vi "TreeEditor.vi"() -> ()   [LabVIEW 2016]
uses:
  ClassDataTree/ClassDataTree.lvclass
panel:
  in  "CreateChild":bool
  in  "LoadToFile":bool
  in  "SaveToFile":bool
  in  "Delete":bool
  in  "Update":bool
  in  "CreateTag":bool
  out "ClassDataTree":refnum<class "ClassDataTree.lvclass">
  in  "ExitApplocation":bool
  out "error out":errorcluster
  in  "CreateNameTag":string
  in  "Tree":string[](tree)
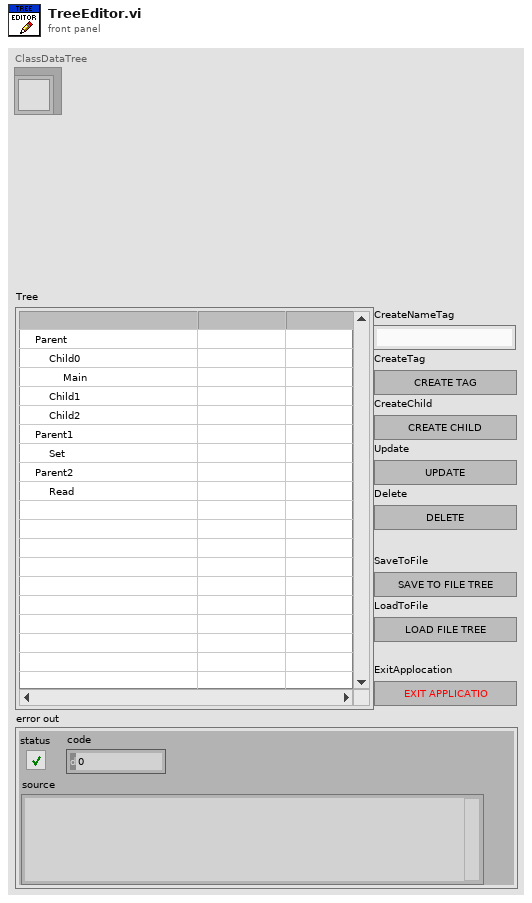
[diagram p1: front panel]
types:
  T1 = typedef "LVPoint32TypeDef.ctl" = cluster{"Horizontal":i32, "Vertical":i32}
  T2 = cluster{"Shift":bool, "Ctrl":bool, "Alt":bool, "Cmd":bool, "Opt":bool}
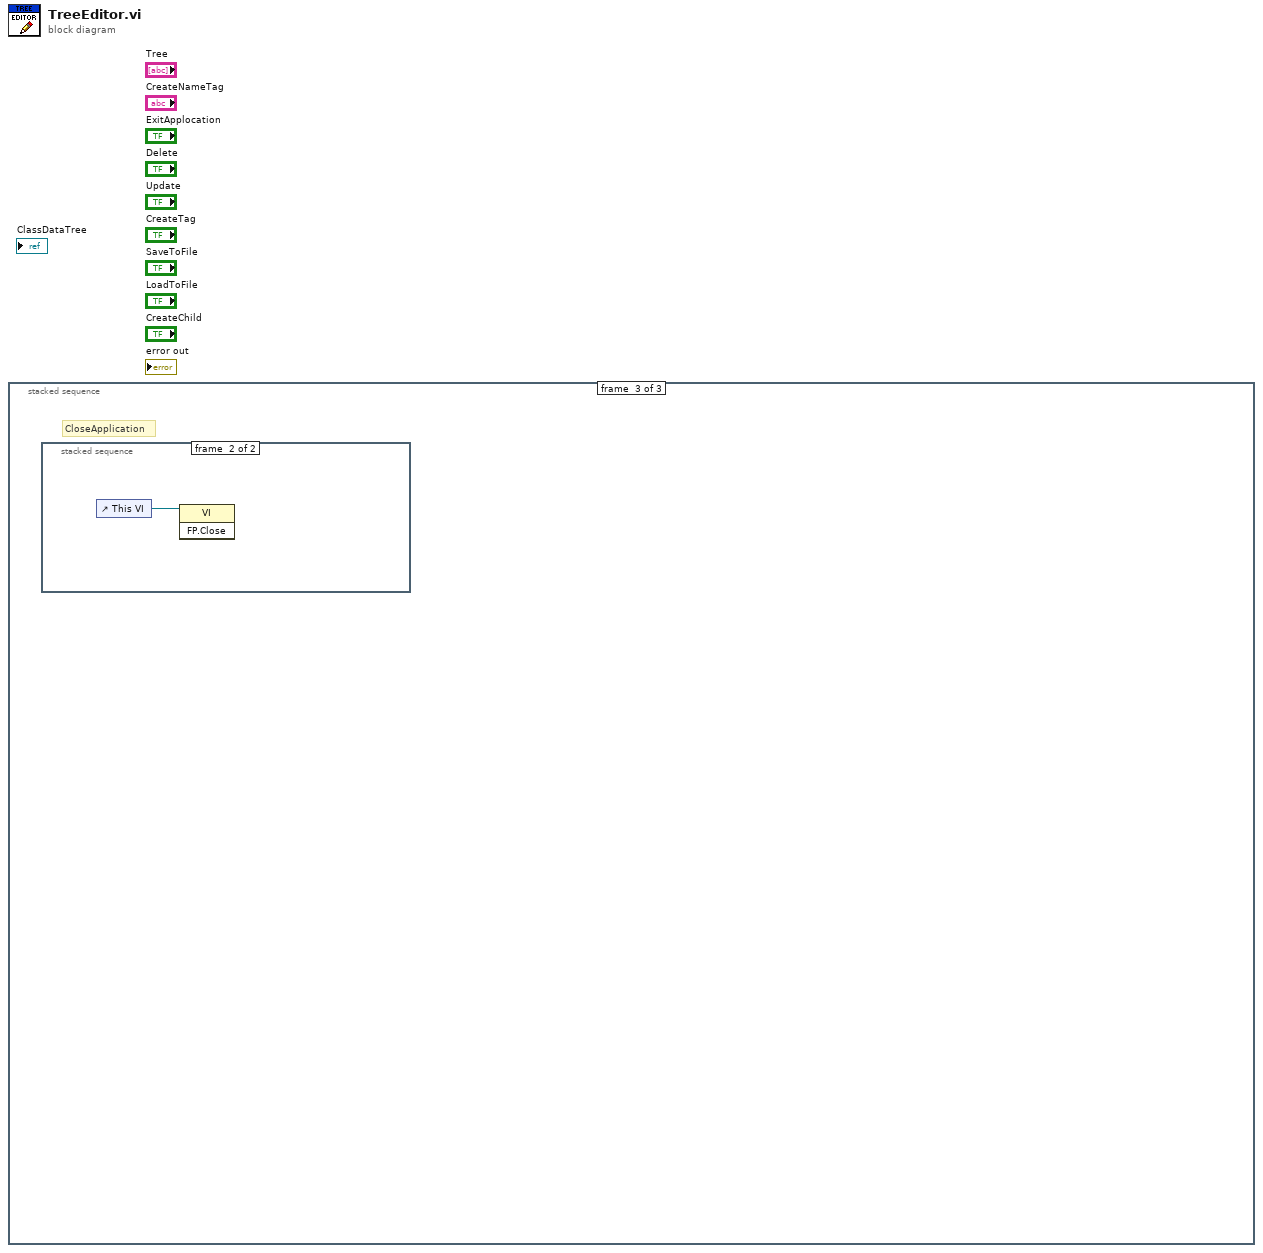
[diagram p0: block diagram]
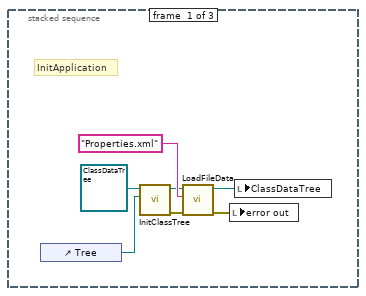
[diagram p2: hidden frame]
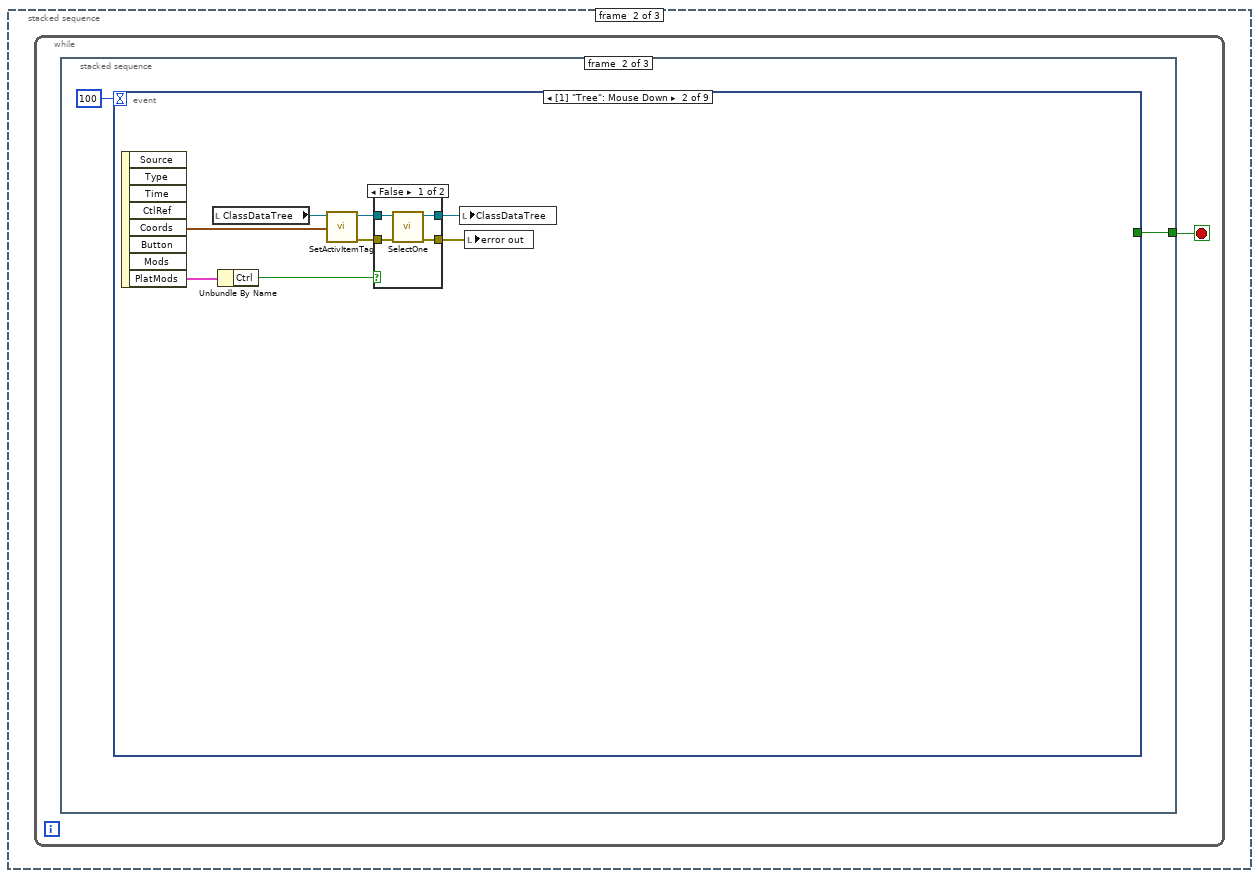
[diagram p3: hidden frame]
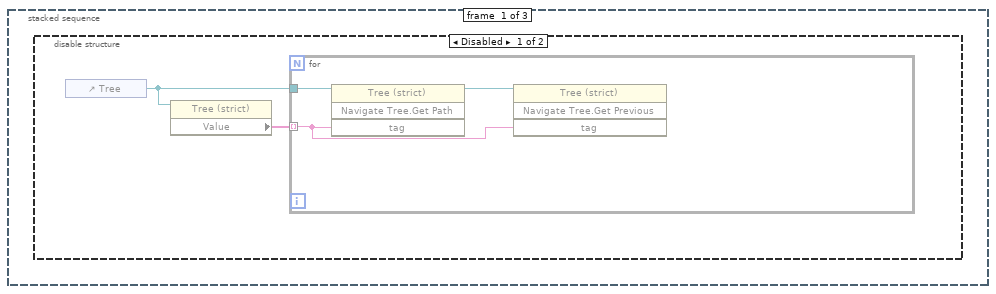
[diagram p4: hidden frame]
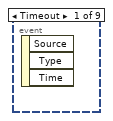
[diagram p6: hidden frame]
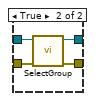
[diagram p7: hidden frame]
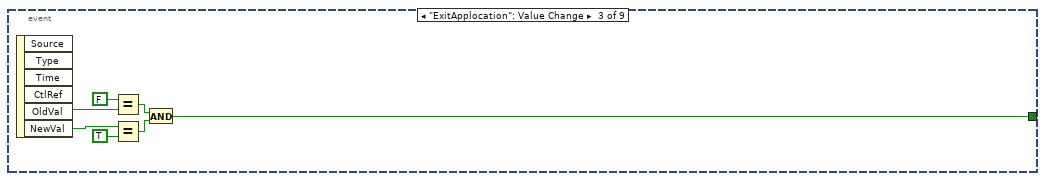
[diagram p8: hidden frame]
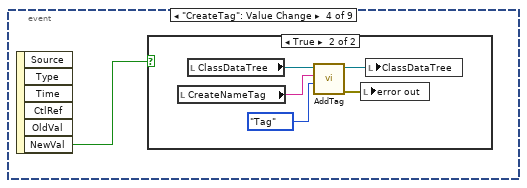
[diagram p9: hidden frame]
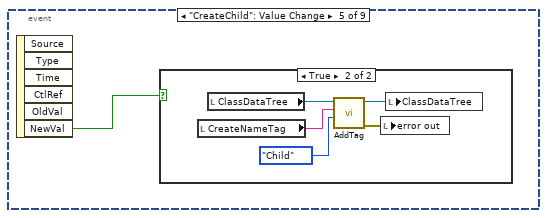
[diagram p11: hidden frame]
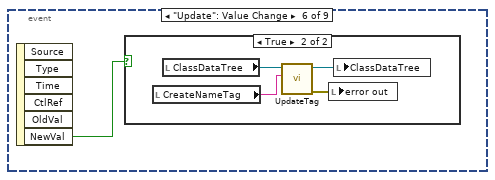
[diagram p13: hidden frame]
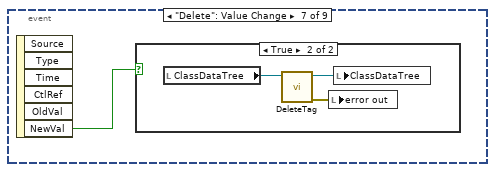
[diagram p15: hidden frame]
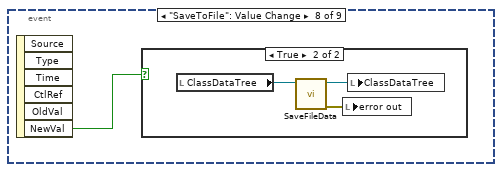
[diagram p17: hidden frame]
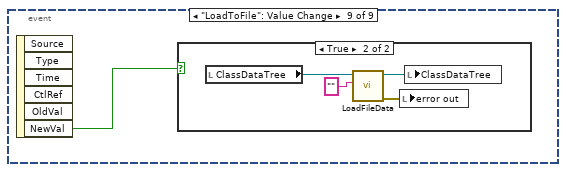
[diagram p19: hidden frame]
diagram:
  n1 = stacked-sequence {
    frame #0 {
      # "InitApplication"
      n2 = control-ref of="Tree"() -> (w1:refnum<vi>)
      n3 = call-dynamic "InitClassTree.vi"("TreeStrict"=w1, "ClassDataTree in"=refnum<class "ClassDataTree.lvclass"> refnum ("ClassDataTree.lvclass")) -> ("error out"=w2:errorcluster, "ClassDataTree out"=w3:refnum<class "ClassDataTree.lvclass">)  [unwired: 8 in]
      n4 = call-dynamic "LoadFileData.vi"("error in (no error)"=w2, "NameFiles"="Properties.xml" ("string"), "ClassDataTree in"=w3) -> ("error out"=w6:errorcluster, "ClassDataTree out"=w7:refnum<class "ClassDataTree.lvclass">)  [unwired: 7 in]
      n5 = local write "error out"(w6) -> ()
      n6 = local write "ClassDataTree"(w7) -> ()
    }
    frame #1 {
      n7 = while {
        stop <- w8 stop-if-true
        n8 = stacked-sequence {
          tunnel: [_ w14 _] -> w8
          frame #0 {
            n9 = disable-structure shown="Disabled" {
              frame Disabled {
                n10 = control-ref of="Tree"() -> (w10:refnum<vi>)
                n11 = property class="Tree (strict)"(reference=w10) -> ("Value"=w9:string[])  [unwired: 1 in, 2 out]
                n12 = for {
                  tunnel: w10 -> [w13]
                  tunnel: w9 -> [w12] mode=indexing
                  n13 = invoke class="Tree (strict)" method="Navigate Tree.Get Path"(reference=w13, "tag"=w12) -> (reference out=w11:refnum<vi>)  [unwired: 2 in, 3 out]
                  n14 = invoke class="Tree (strict)" method="Navigate Tree.Get Previous"(reference=w11, "tag"=w12) -> ()  [unwired: 2 in, 4 out]
                }
              }
              frame Enabled {
              }
            }
          }
          frame #1 {
            n15 = event shown="[1] \"Tree\": Mouse Down" {
              selector: _ -> [_ _ _ _ _ _ _ _ _]
              dyn-events: _ -> [_ _ _ _ _ _ _ _ _]
              timeout: 100 -> [_ _ _ _ _ _ _ _ _]
              tunnel: [_ _ w32 _ _ _ _ _ _] -> w14
              event Timeout {
                n16 = event-data() -> ()  [unwired: 1 in, 3 out]
              }
              event "Tree": Mouse Down {
                n17 = event-data() -> ("Coords"=w19:T1, "PlatMods"=w23:T2)  [unwired: 1 in, 6 out]
                n18 = local read "ClassDataTree"() -> (w20:refnum<class "ClassDataTree.lvclass">)
                n19 = Unbundle By Name(w23) -> ("Ctrl"=w22:bool)
                n20 = call-dynamic "SetActivItemTag.vi"("Coords"=w19, "ClassDataTree in"=w20) -> ("error out"=w17:errorcluster, "ClassDataTree out"=w18:refnum<class "ClassDataTree.lvclass">)  [unwired: 8 in]
                n21 = case shown="False" w22 {
                  tunnel: [w27 w29] -> w21
                  tunnel: w18 -> [w26 w31]
                  tunnel: w17 -> [w25 w30]
                  tunnel: [w24 w28] -> w16
                  frame False {
                    n22 = call-dynamic "SelectOne.vi"("error in (no error)"=w25, "ClassDataTree in"=w26) -> ("error out"=w24:errorcluster, "ClassDataTree out"=w27:refnum<class "ClassDataTree.lvclass">)  [unwired: 8 in]
                  }
                  frame True {
                    n23 = call-dynamic "SelectGroup.vi"("error in (no error)"=w30, "ClassDataTree in"=w31) -> ("error out"=w28:errorcluster, "ClassDataTree out"=w29:refnum<class "ClassDataTree.lvclass">)  [unwired: 8 in]
                  }
                }
                n24 = local write "ClassDataTree"(w21) -> ()
                n25 = local write "error out"(w16) -> ()
              }
              event "ExitApplocation": Value Change {
                n26 = event-data() -> ("OldVal"=w36:bool, "NewVal"=w38:bool)  [unwired: 1 in, 4 out]
                n27 = Equal?(x=FALSE, y=w36) -> (x = y?=w34:bool)
                n28 = Equal?(x=w38, y=TRUE) -> (x = y?=w33:bool)
                n29 = And(x=w34, y=w33) -> (x .and. y?=w32:bool)
              }
              event "CreateTag": Value Change {
                n30 = event-data() -> ("NewVal"=w39:bool)  [unwired: 1 in, 5 out]
                n31 = case shown="True" w39 {
                  frame False {
                  }
                  frame True {
                    n32 = local read "CreateNameTag"() -> (w42:string)
                    n33 = local read "ClassDataTree"() -> (w44:refnum<class "ClassDataTree.lvclass">)
                    n34 = call-dynamic "AddTag.vi"("TupeTerminode"=enum16{"Tag", "Child"}."Tag" ("Enum"), "CreateNameTag"=w42, "ClassDataTree in"=w44) -> ("error out"=w41:errorcluster, "ClassDataTree out"=w43:refnum<class "ClassDataTree.lvclass">)  [unwired: 7 in]
                    n35 = local write "error out"(w41) -> ()
                    n36 = local write "ClassDataTree"(w43) -> ()
                  }
                }
              }
              event "CreateChild": Value Change {
                n37 = event-data() -> ("NewVal"=w45:bool)  [unwired: 1 in, 5 out]
                n38 = case shown="True" w45 {
                  frame False {
                  }
                  frame True {
                    n39 = local read "CreateNameTag"() -> (w48:string)
                    n40 = local read "ClassDataTree"() -> (w50:refnum<class "ClassDataTree.lvclass">)
                    n41 = call-dynamic "AddTag.vi"("TupeTerminode"=enum16{"Tag", "Child"}."Child" ("Enum"), "CreateNameTag"=w48, "ClassDataTree in"=w50) -> ("error out"=w47:errorcluster, "ClassDataTree out"=w49:refnum<class "ClassDataTree.lvclass">)  [unwired: 7 in]
                    n42 = local write "error out"(w47) -> ()
                    n43 = local write "ClassDataTree"(w49) -> ()
                  }
                }
              }
              event "Update": Value Change {
                n44 = event-data() -> ("NewVal"=w51:bool)  [unwired: 1 in, 5 out]
                n45 = case shown="True" w51 {
                  frame False {
                  }
                  frame True {
                    n46 = local read "CreateNameTag"() -> (w52:string)
                    n47 = local read "ClassDataTree"() -> (w55:refnum<class "ClassDataTree.lvclass">)
                    n48 = call-dynamic "UpdateTag.vi"("CreateNameTag"=w52, "ClassDataTree in"=w55) -> ("error out"=w53:errorcluster, "ClassDataTree out"=w54:refnum<class "ClassDataTree.lvclass">)  [unwired: 8 in]
                    n49 = local write "error out"(w53) -> ()
                    n50 = local write "ClassDataTree"(w54) -> ()
                  }
                }
              }
              event "Delete": Value Change {
                n51 = event-data() -> ("NewVal"=w56:bool)  [unwired: 1 in, 5 out]
                n52 = case shown="True" w56 {
                  frame False {
                  }
                  frame True {
                    n53 = local read "ClassDataTree"() -> (w58:refnum<class "ClassDataTree.lvclass">)
                    n54 = call-dynamic "DeleteTag.vi"("ClassDataTree in"=w58) -> ("error out"=w57:errorcluster, "ClassDataTree out"=w59:refnum<class "ClassDataTree.lvclass">)  [unwired: 9 in]
                    n55 = local write "error out"(w57) -> ()
                    n56 = local write "ClassDataTree"(w59) -> ()
                  }
                }
              }
              event "SaveToFile": Value Change {
                n57 = event-data() -> ("NewVal"=w60:bool)  [unwired: 1 in, 5 out]
                n58 = case shown="True" w60 {
                  frame False {
                  }
                  frame True {
                    n59 = local read "ClassDataTree"() -> (w63:refnum<class "ClassDataTree.lvclass">)
                    n60 = call-dynamic "SaveFileData.vi"("ClassDataTree in"=w63) -> ("error out"=w61:errorcluster, "ClassDataTree out"=w62:refnum<class "ClassDataTree.lvclass">)  [unwired: 9 in]
                    n61 = local write "error out"(w61) -> ()
                    n62 = local write "ClassDataTree"(w62) -> ()
                  }
                }
              }
              event "LoadToFile": Value Change {
                n63 = event-data() -> ("NewVal"=w64:bool)  [unwired: 1 in, 5 out]
                n64 = case shown="True" w64 {
                  frame False {
                  }
                  frame True {
                    n65 = local read "ClassDataTree"() -> (w66:refnum<class "ClassDataTree.lvclass">)
                    n66 = call-dynamic "LoadFileData.vi"("NameFiles"="", "ClassDataTree in"=w66) -> ("error out"=w67:errorcluster, "ClassDataTree out"=w68:refnum<class "ClassDataTree.lvclass">)  [unwired: 8 in]
                    n67 = local write "error out"(w67) -> ()
                    n68 = local write "ClassDataTree"(w68) -> ()
                  }
                }
              }
            }
          }
          frame #2 {
          }
        }
      }
    }
    frame #2 {
      # "CloseApplication"
      n69 = stacked-sequence {
        frame #0 {
          n70 = local read "ClassDataTree"() -> (w72:refnum<class "ClassDataTree.lvclass">)
          n71 = call-dynamic "SaveFileData.vi"("NameFile"="Properties.xml" ("string"), "ClassDataTree in"=w72) -> ("error out"=w70:errorcluster, "ClassDataTree out"=w71:refnum<class "ClassDataTree.lvclass">)  [unwired: 8 in]
          n72 = local write "error out"(w70) -> ()
          n73 = local write "ClassDataTree"(w71) -> ()
        }
        frame #1 {
          n74 = control-ref of="This VI"() -> (w73:refnum<vi>)
          n75 = invoke class="VI" method="FP.Close"(reference=w73) -> ()  [unwired: 2 in, 3 out]
        }
      }
    }
  }
